vi "getSerializedData.vi"(0 "reference":refnum<class "ClassRelationshipEdge.lvclass">, 5 "error in (no error)":errorcluster) -> (14 "reference out":refnum<class "ClassRelationshipEdge.lvclass">, 15 "startNode":refnum<class "AbstractNode.lvclass">, 16 "endNode":refnum<class "AbstractNode.lvclass">, 17 "xmlOut":string, 19 "error out":errorcluster)   [LabVIEW 2020, in "ClassRelationshipEdge.lvclass"]
uses:
  <resource>/Framework/Providers/Open_GDS/UML/ClassRelationshipEdge_class/ClassRelationshipEdge.lvclass
  C:/Program Files (x86)/National Instruments/LabVIEW 2020/resource/Framework/Providers/Open_GDS/UML/SegmentedLineEdge_class/SegmentedLineEdge.lvclass
  C:/Program Files (x86)/National Instruments/LabVIEW 2020/resource/Framework/Providers/Open_GDS/UML/AbstractEdge_class/AbstractEdge.lvclass
  <resource>/Framework/Providers/Open_GDS/UML/AbstractNode_class/AbstractNode.lvclass
  <resource>/Framework/Providers/Open_GDS/UML/General/Point/Point Point2D.ctl
  <resource>/Framework/Providers/Open_GDS/UML/ArrowHead_class/ArrowHead.lvclass
  <resource>/Framework/Providers/Open_GDS/UML/BentStyle_class/BentStyle.lvclass
  <resource>/Framework/Providers/Open_GDS/UML/LineStyle_class/LineStyle.lvclass
  <resource>/Framework/Providers/Open_GDS/UML/SegmentedLineEdge_class/SegmentedLineEdge.lvclass
  <resource>/Framework/Providers/Open_GDS/UML/AbstractEdge_class/AbstractEdge.lvclass
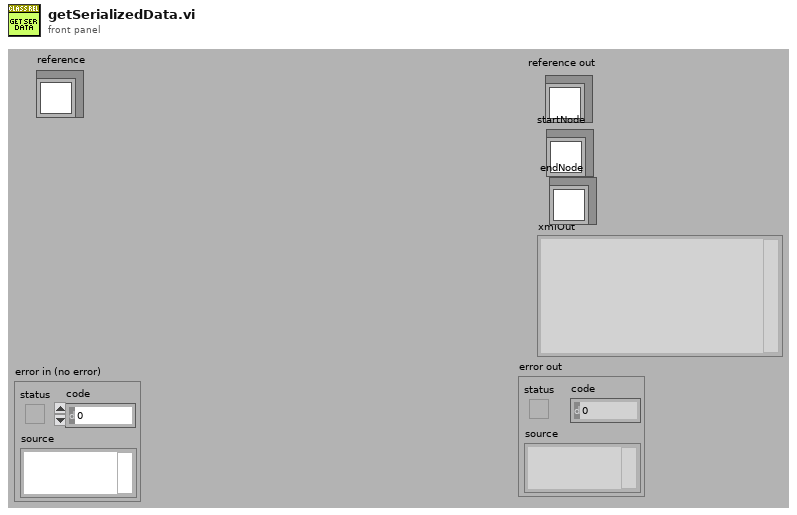
[diagram p1: front panel]
types:
  T1 = typedef "Point Point2D.ctl" = cluster{"x":dbl, "y":dbl}
  T2 = cluster{"Base class":cluster{"Base class":cluster{"Base class":cluster{"start":refnum<k1>, "end":refnum<k1>}}, "lineStyle":refnum<k1>, "startArrowHead":refnum<k1>, "endArrowHead":refnum<k1>, "startLabel":string, "midLabel":string, "endLabel":string, "MidLabelOffset":T1, "SplitWire":bool}, "bentStyleRef":refnum<k1>, "startConnectionOffset":cluster{"x":i32, "y":i32}, "endConnectionOffset":cluster{"x":i32, "y":i32}, "MidLineOffset":cluster{"x":i32, "y":i32}, "DepClass":cluster{"ThisVIs/Ctls":path[], "Dependent_VIs/Ctls":path[]}}
  T3 = typedef "ClassRelationshipEdge.lvclass/ObjectAttributes.ctl" = cluster{"bentStyleRef":refnum<class "BentStyle.lvclass">, "startConnectionOffset":cluster{"x":i32, "y":i32}, "endConnectionOffset":cluster{"x":i32, "y":i32}, "MidLineOffset":cluster{"x":i32, "y":i32}, "DepClass":T4}
  T4 = typedef "ReversedEngineering_ViDependencyDetailsType.ctl" = cluster{"ThisVIs/Ctls":path[], "Dependent_VIs/Ctls":path[]}
  T5 = typedef "SegmentedLineEdge.lvclass/ObjectAttributes.ctl" = cluster{"lineStyle":refnum<class "LineStyle.lvclass">, "startArrowHead":refnum<class "ArrowHead.lvclass">, "endArrowHead":refnum<class "ArrowHead.lvclass">, "startLabel":string, "midLabel":string, "endLabel":string, "MidLabelOffset":T1, "SplitWire":bool}
  T6 = typedef "AbstractEdge.lvclass/ObjectAttributes.ctl" = cluster{"start":refnum<class "AbstractNode.lvclass">, "end":refnum<class "AbstractNode.lvclass">}
  T7 = cluster{"Attributes":cluster{"Base class":cluster{"Base class":cluster{"Base class":cluster{"start":refnum<k1>, "end":refnum<k1>}}, "lineStyle":refnum<k1>, "startArrowHead":refnum<k1>, "endArrowHead":refnum<k1>, "startLabel":string, "midLabel":string, "endLabel":string, "MidLabelOffset":T1, "SplitWire":bool}, "bentStyleRef":refnum<k1>, "startConnectionOffset":cluster{"x":i32, "y":i32}, "endConnectionOffset":cluster{"x":i32, "y":i32}, "MidLineOffset":cluster{"x":i32, "y":i32}, "DepClass":cluster{"ThisVIs/Ctls":path[], "Dependent_VIs/Ctls":path[]}}, "Type(String)":string, "Object name":string, "Object name":string, "Object name":string}
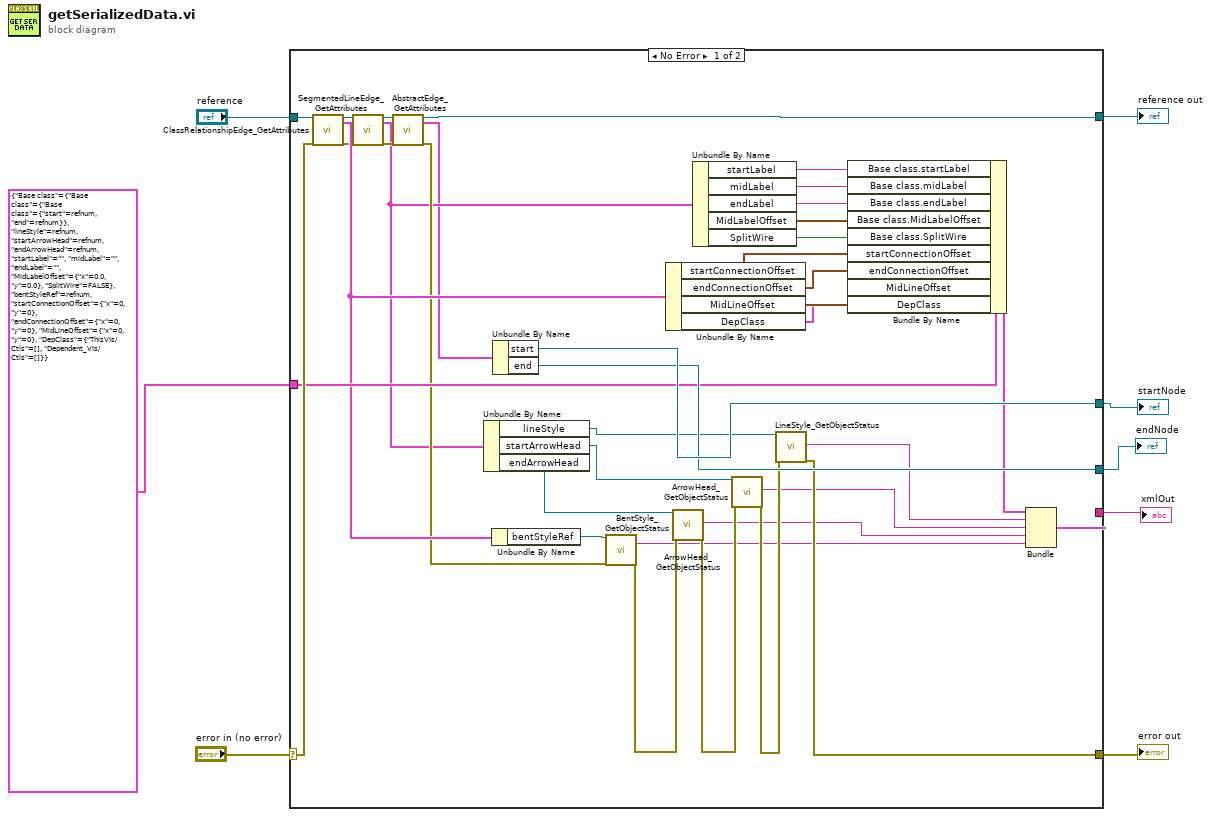
[diagram p0: block diagram]
diagram:
  n1 = case shown="No Error" "error in (no error)" {
    selector: "error in (no error)" -> [w46 w47]
    tunnel: "reference" -> [w45 w48]
    tunnel: [w33 w47] -> w6
    tunnel: [w15 w48] -> w5
    tunnel: [w43 _] -> w4
    tunnel: [w42 _] -> w3
    tunnel: [w41 _] -> w2
    tunnel: T2 {"Base class"={"Base class"={"Base class"={"start"=refnum, "end"=refnum}}, "lineStyle"=refnum, "startArrowHead"=refnum, "endArrowHead"=refnum, "startLabel"="", "midLabel"="", "endLabel"="", "MidLabelOffset"={"x"=0.0, "y"=0.0}, "SplitWire"=FALSE}, "bentStyleRef"=refnum, "startConnectionOffset"={"x"=0, "y"=0}, "endConnectionOffset"={"x"=0, "y"=0}, "MidLineOffset"={"x"=0, "y"=0}, "DepClass"={"ThisVIs/Ctls"=[], "Dependent_VIs/Ctls"=[]}} ("Attributes") -> [w32 _]
    frame No Error {
      n2 = call <resource>:"ClassRelationshipEdge_GetAttributes.vi"("reference in"=w45, "error in (no error)"=w46) -> ("reference out"=w20:refnum<class "ClassRelationshipEdge.lvclass">, "Data"=w21:T3, "error out"=w19:errorcluster)  [unwired: 1 in, 14 out]
      n3 = call <resource>:"SegmentedLineEdge_GetAttributes.vi"("reference in"=w20, "error in (no error)"=w19) -> ("reference out"=w18:refnum<class "ClassRelationshipEdge.lvclass">, "Data"=w14:T5, "error out"=w17:errorcluster)  [unwired: 14 in, 1 out]
      n4 = call <resource>:"AbstractEdge_GetAttributes.vi"("reference in"=w18, "error in (no error)"=w17) -> ("reference out"=w15:refnum<class "ClassRelationshipEdge.lvclass">, "Data"=w13:T6, "error out"=w16:errorcluster)  [unwired: 14 in, 1 out]
      n5 = Unbundle By Name(w14) -> ("lineStyle"=w40:refnum<class "LineStyle.lvclass">, "startArrowHead"=w39:refnum<class "ArrowHead.lvclass">, "endArrowHead"=w38:refnum<class "ArrowHead.lvclass">)
      n6 = Unbundle By Name(w21) -> ("bentStyleRef"=w37:refnum<class "BentStyle.lvclass">)
      n7 = Unbundle By Name(w13) -> ("start"=w42:refnum<class "AbstractNode.lvclass">, "end"=w41:refnum<class "AbstractNode.lvclass">)
      n8 = call <resource>:"BentStyle_GetObjectStatus.vi"("reference in"=w37, "error in (no error)"=w16) -> ("Object name"=w9:string, "error out"=w36:errorcluster)  [unwired: 1 in, 15 out]
      n9 = Unbundle By Name(w21) -> ("startConnectionOffset"=w25:cluster{"x":i32, "y":i32}, "endConnectionOffset"=w24:cluster{"x":i32, "y":i32}, "MidLineOffset"=w23:cluster{"x":i32, "y":i32}, "DepClass"=w22:T4)
      n10 = call <resource>:"ArrowHead_GetObjectStatus.vi"("reference in"=w38, "error in (no error)"=w36) -> ("Object name"=w10:string, "error out"=w35:errorcluster)  [unwired: 1 in, 15 out]
      n11 = Unbundle By Name(w14) -> ("startLabel"=w30:string, "midLabel"=w29:string, "endLabel"=w28:string, "MidLabelOffset"=w27:T1, "SplitWire"=w26:bool)
      n12 = call <resource>:"ArrowHead_GetObjectStatus.vi"("reference in"=w39, "error in (no error)"=w35) -> ("Object name"=w11:string, "error out"=w34:errorcluster)  [unwired: 1 in, 15 out]
      n13 = call <resource>:"LineStyle_GetObjectStatus.vi"("reference"=w40, "error in (no error)"=w34) -> ("Type(String)"=w12:string, "error out"=w33:errorcluster)  [unwired: 15 in, 1 out]
      n14 = Bundle By Name(cluster=w32, "Base class.startLabel"=w30, "Base class.midLabel"=w29, "Base class.endLabel"=w28, "Base class.MidLabelOffset"=w27, "Base class.SplitWire"=w26, "startConnectionOffset"=w25, "endConnectionOffset"=w24, "MidLineOffset"=w23, "DepClass"=w22) -> (w31:T2)
      n15 = Bundle("Attributes"=w31, "Type(String)"=w12, "Object name"=w11, "Object name"=w10, "Object name"=w9) -> (w44:T7)  [unwired: 1 out]
      n16 = Flatten To XML(6:w44) -> (2:w43:string)
    }
    frame Error {
    }
  }
  "reference out" <- w5
  "error out" <- w6
  "startNode" <- w3
  "endNode" <- w2
  "xmlOut" <- w4
